vi "CRYSet Probe Curve Front Panel.vi"(11 "Vi Ref":refnum<vi>) -> ()   [LabVIEW 2013]
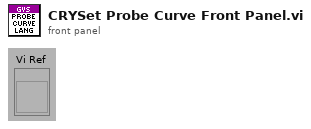
[diagram p1: front panel]
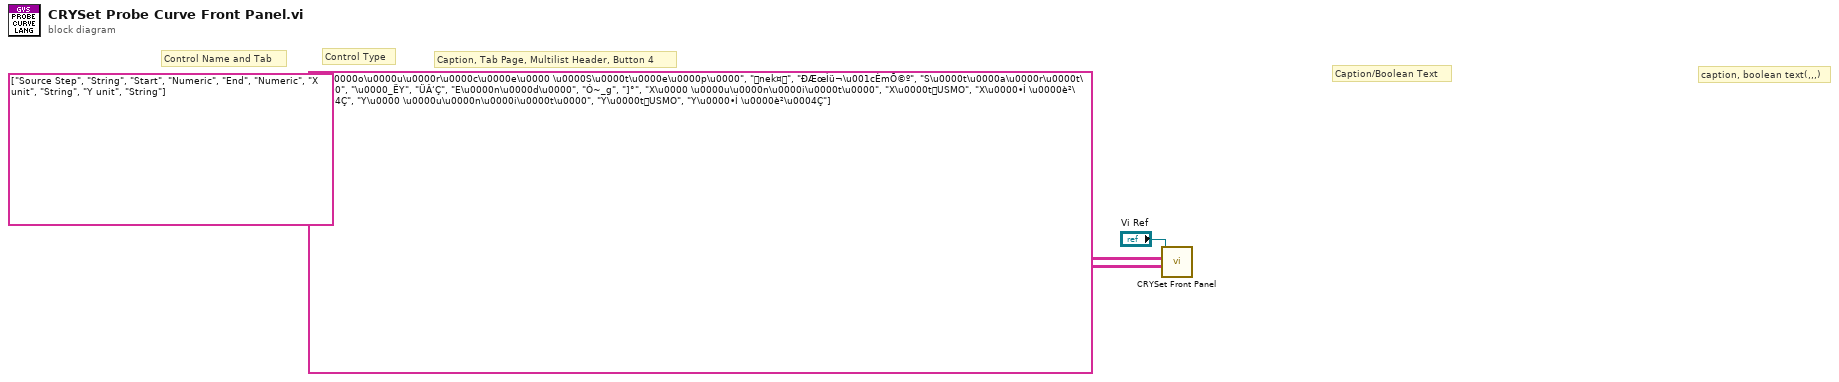
[diagram p0: block diagram]
diagram:
  # "Caption, Tab Page, Multilist Header, Button 4"
  # "Control Type"
  # "Control Name and Tab"
  # "caption, boolean text(,,,)"
  # "Caption/Boolean Text"
  n1 = call "CRYSet Front Panel.vi"("Caption(Boolean Text)"=string[][] [["S\u0000o\u0000u\u0000r\u0000c\u0000e\u0000 \u0000S\u0000t\u0000e\u0000p\u0000", "nek¤", "ÐÆœÌü¬\u001cÈmÕ©º"], ["S\u0000t\u0000a\u0000r\u0000t\u0000", "\u0000_ËY", "ÜÂ‘Ç"], ["E\u0000n\u0000d\u0000", "Ó~_g", "]°"], ["X\u0000 \u0000u\u0000n\u0000i\u0000t\u0000", "X\u0000tUSMO", "X\u0000•Í \u0000è²\u0004Ç"], ["Y\u0000 \u0000u\u0000n\u0000i\u0000t\u0000", "Y\u0000tUSMO", "Y\u0000•Í \u0000è²\u0004Ç"]], "Control ID and Type(Label Name, Type)"=string[][] [["Source Step", "String"], ["Start", "Numeric"], ["End", "Numeric"], ["X unit", "String"], ["Y unit", "String"]], "Vi Ref"="Vi Ref") -> ()  [unwired: 9 in]
